vi "Align Visualizer v2.vi"(0 "Trajectory Data":T1, 1 "Points":cluster{"x":dbl, "y":dbl, "th":dbl}[](array[cluster]), 2 "Picture in":refnum<vi>, 3 "Sample Period (s)":dbl=0.02 min=0.001 max=1.0 format="%#_6p", 4 "Time (s)":dbl(slide) scale=0.0..4.32 scale format="%#.1g") -> (5 "Picture":picture)   [LabVIEW 2023]
uses:
  bordeaux-pathinator/Bordeaux/Types/Trajectory Data.ctl
  bordeaux-pathinator/Bordeaux/Types/Segment Type.ctl
  bordeaux-pathinator/Bordeaux/Types/Single Cmd Info.ctl
  <vilib>/picture/picture.llb/imagedata.ctl
panel:
  out "new picture":picture
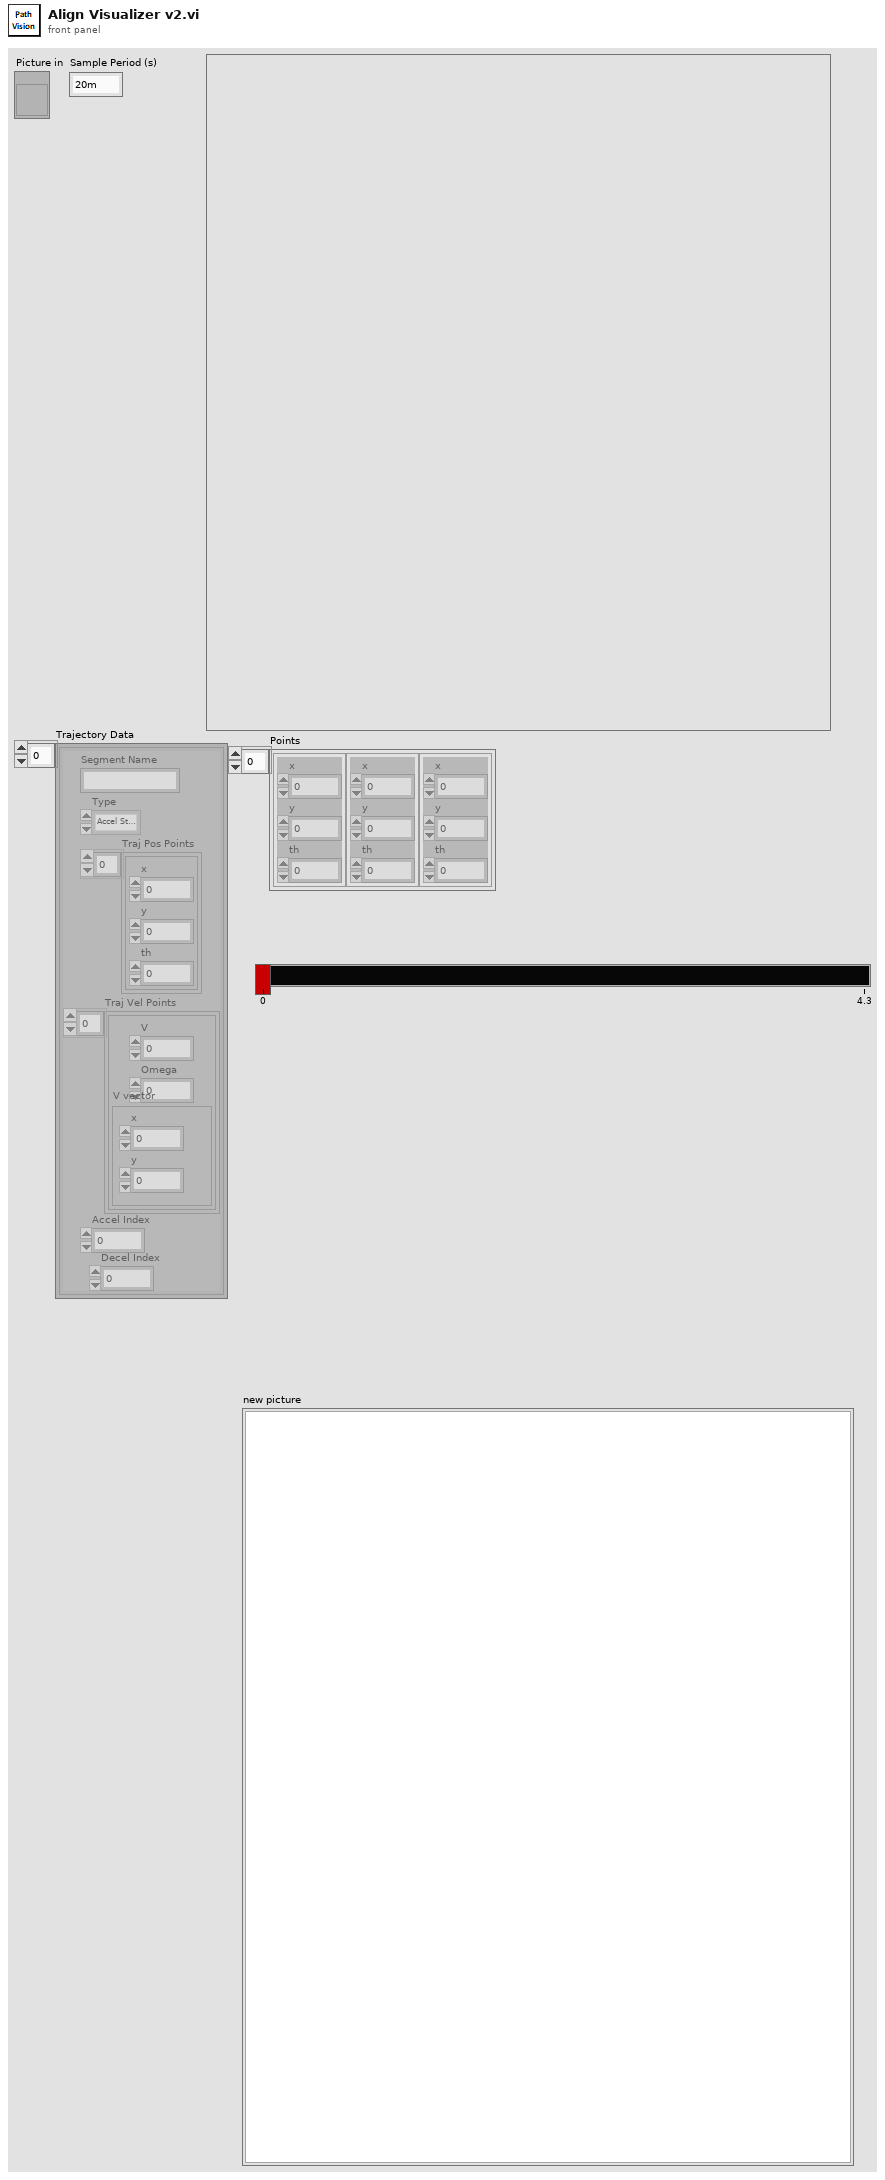
[diagram p1: front panel]
types:
  T1 = typedef "Trajectory Data.ctl" = cluster{"Segment Name":string, "Type":T2, "Traj Pos Points":cluster{"x":dbl, "y":dbl, "th":dbl}[], "Traj Vel Points":cluster{"V":dbl, "Omega":dbl, "V vector":cluster{"y":dbl, "x":dbl}}[], "Accel Index":i32, "Decel Index":i32}[]
  T2 = typedef "Segment Type.ctl" = enum16{"Accel Straight", "Const Straight", "Blend", "Circle", "Bezier"}
  T3 = typedef "Single Cmd Info.ctl" = cluster{"Name":string, "CPTM.DataType":variant, "All Control Values Variant":cluster{"Name":string, "Variant Data":variant}[], "icon full":T4, "icon scaled":T4, "Path":path, "Subsystem Color":u32}
  T4 = typedef "imagedata.ctl" = cluster{"image type":i32, "image depth":i32, "image":u8[], "mask":u8[], "colors":u32[], "Rectangle":cluster{"left":i16, "top":i16, "right":i16, "bottom":i16}}
  T5 = cluster{"Index":i32, "Pt Test Results":enum16{"Miss", "Rect Hit", "Arrow Hit"}}
  T6 = cluster{"Horizontal":dbl, "Vertical":dbl, "th":dbl}
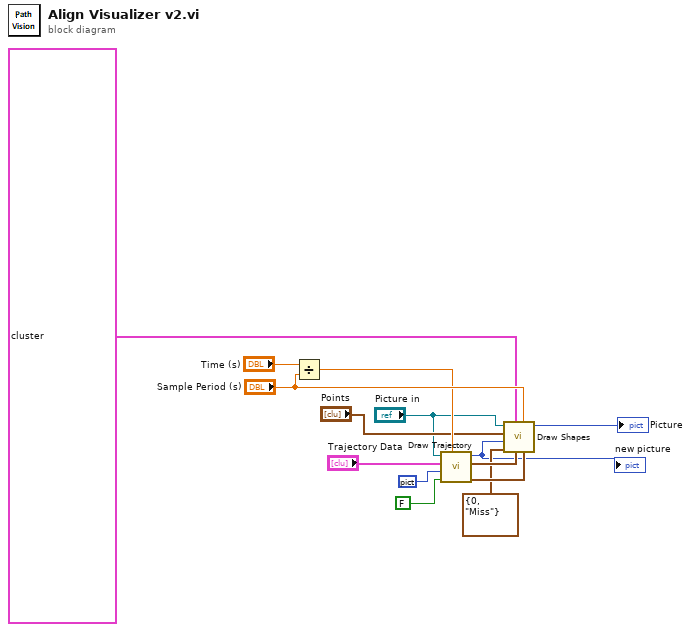
[diagram p0: block diagram]
diagram:
  n1 = Divide(x="Time (s)", y="Sample Period (s)") -> (x/y=w6:dbl)
  n2 = call "Draw Trajectory.vi"("Robot Index"=w6, "Hide Path"=FALSE, "new picture in"=picture data[5B] ("new picture"), "Trajectory Data"="Trajectory Data", "Picture in"="Picture in") -> ("Path Points"=w11:cluster{"x":dbl, "y":dbl}[], "Output Point"=w13:T6, "new picture"=w1:picture)  [unwired: 4 in]
  "new picture" <- w1
  n3 = call "Draw Shapes.vi"("Path Points"=w11, "Sample Period (s)"="Sample Period (s)", "Output Point"=w13, "Commands"=cluster{"Time (s)":dbl, T3, "Enabled":bool}[] [{"Time (s)"=0.0, {"Name"="", "CPTM.DataType"=variant, "All Control Values Variant"=[], "icon full"={"image type"=0, "image depth"=0, "image"=[], "mask"=[], "colors"=[], "Rectangle"={"left"=0, "top"=0, "right"=0, "bottom"=0}}, "icon scaled"={"image type"=0, "image depth"=0, "image"=[], "mask"=[], "colors"=[], "Rectangle"={"left"=0, "top"=0, "right"=0, "bottom"=0}}, "Path"=path "", "Subsystem Color"=16777216}, "Enabled"=FALSE}], "Results"=T5 {"Index"=0, "Pt Test Results"=enum."Miss"}, "new picture in"=w1, "Points"="Points", "Picture in"="Picture in") -> ("new picture out"=→"Picture":picture)  [unwired: 3 in]
